vi "1d to boolean sub vi.vi"(1 "A":dbl min=-9.0 max=9.0 step=1.0) -> (0 "initialized array":bool[](array[boolean]))   [LabVIEW 2020]
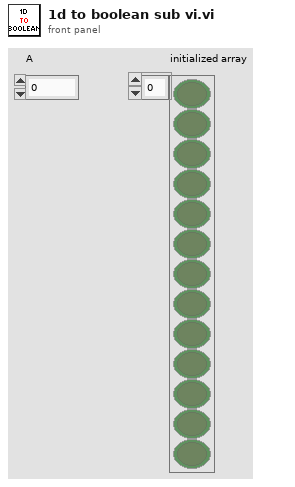
[diagram p1: front panel]
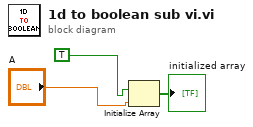
[diagram p0: block diagram]
diagram:
  n1 = Initialize Array(TRUE, "A") -> (→"initialized array":bool[])
